vi "Drivetrain.vi"(10 "Duration":i64, 11 "rt fifo":refnum<k33>) -> ()   [LabVIEW 2015]
uses:
  Drive Metrics.ctl
  Drive States.ctl
  Copilot States.ctl
panel:
  in  "Drive Metrics":T1
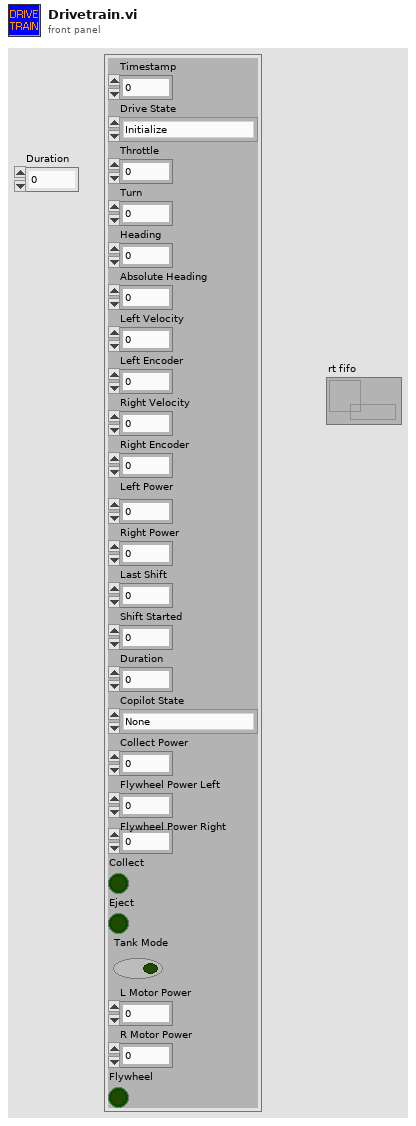
[diagram p1: front panel]
types:
  T1 = typedef "Drive Metrics.ctl" = cluster{"Timestamp":u32, "Drive State":T2, "Throttle":dbl, "Turn":dbl, "Heading":dbl, "Absolute Heading":dbl, "Left Velocity":dbl, "Left Encoder":dbl, "Right Velocity":dbl, "Right Encoder":dbl, "Left Power":dbl, "Right Power":dbl, "Last Shift":u32, "Shift Started":u32, "Duration":i64, "Copilot State":T3, "Collect Power":dbl, "Flywheel Power Left":dbl, "Flywheel Power Right":dbl, "Collect":bool, "Eject":bool, "Tank Mode":bool, "L Motor Power":dbl, "R Motor Power":dbl, "Flywheel":bool}
  T2 = typedef "Drive States.ctl" = enum16{"Initialize", "Low Gear", "Up Shift Begin", "Up Shifting", "Up Shift Delay", "High Gear", "Down Shift Begin", "Down Shifting", "Down Shift Delay"}
  T3 = typedef "Copilot States.ctl" = enum16{"None", "Lift collector", "Boulder to shooter", "Lifting collector", "Lifted Collector", "Collected", "Collecting", "Ejecting", "Dropping arm", "Boulder ready", "Shooter to angle", "Flywheel spin up", "Drop arm", "Flywheel ready"}
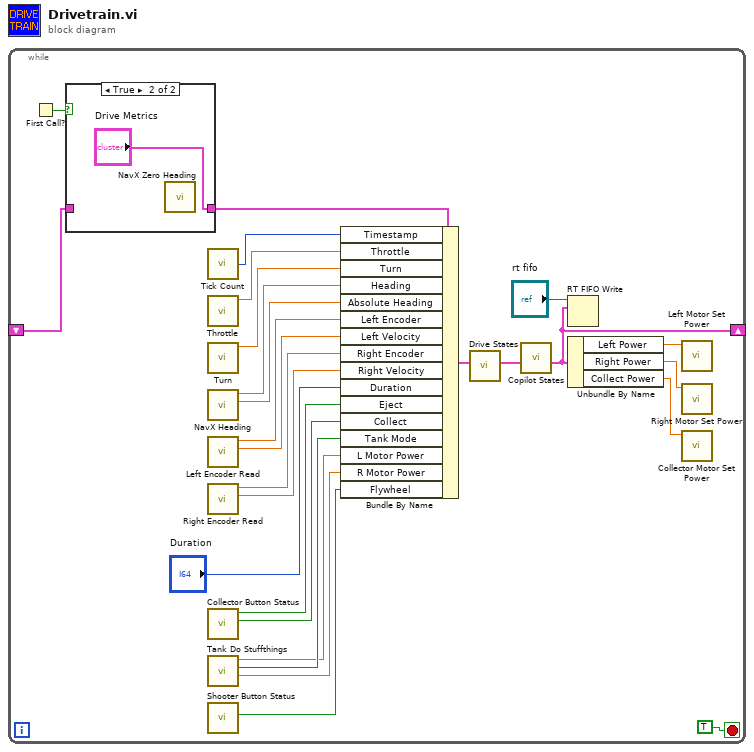
[diagram p0: block diagram]
diagram:
  n1 = while {
    shift-right: [w8] -> _
    shift-left: _ -> [w12]
    stop <- TRUE stop-if-true
    n2 = First Call?() -> (First Call?: T/F=w14:bool)
    n3 = case shown="True" w14 {
      tunnel: [w28 "Drive Metrics"] -> w13
      tunnel: w12 -> [w28 _]
      frame False {
      }
      frame True {
        n4 = call "NavX Zero Heading.vi"() -> ()  [unwired: 11 in, 1 out]
      }
    }
    n5 = call "Tick Count"() -> ("Tick Count(uSec)"=w10:u32)
    n6 = call "Throttle.vi"() -> ("throttle"=w26:dbl)  [unwired: 10 in, 1 out]
    n7 = call "Turn.vi"() -> ("turn"=w25:dbl)  [unwired: 10 in, 1 out]
    n8 = call "NavX Heading.vi"() -> ("Absolute Heading"=w17:dbl, "Heading"=w22:dbl)  [unwired: 9 in, 1 out]
    n9 = call "Left Encoder Read.vi"() -> ("Rate"=w16:dbl, "Distance"=w20:dbl)  [unwired: 7 in, 3 out]
    n10 = call "Right Encoder Read.vi"() -> ("Rate"=w15:dbl, "Distance"=w21:dbl)  [unwired: 7 in, 3 out]
    n11 = call "Collector Button Status.vi"() -> ("Collect"=w5:bool, "Eject"=w6:bool)  [unwired: 9 in, 1 out]
    n12 = call "Tank Do Stuffthings.vi"() -> ("R Motor Power"=w2:dbl, "Tank Mode"=w4:bool, "L Motor Power"=w3:dbl)  [unwired: 8 in, 1 out]
    n13 = call "Shooter Button Status.vi"() -> ("Flywheel"=w1:bool)  [unwired: 10 in, 1 out]
    n14 = Bundle By Name(cluster=w13, "Timestamp"=w10, "Throttle"=w26, "Turn"=w25, "Heading"=w22, "Absolute Heading"=w17, "Left Encoder"=w20, "Left Velocity"=w16, "Right Encoder"=w21, "Right Velocity"=w15, "Duration"="Duration", "Eject"=w6, "Collect"=w5, "Tank Mode"=w4, "L Motor Power"=w3, "R Motor Power"=w2, "Flywheel"=w1) -> (w18:T1)
    n15 = call "Drive States.vi"("Drive Metrics in"=w18) -> ("Drive Metrics out"=w9:T1)  [unwired: 10 in]
    n16 = call "Copilot States.vi"("Drive Metrics in"=w9) -> ("Drive Metrics out"=w8:T1)  [unwired: 10 in]
    n17 = RT FIFO Write(0:"rt fifo", 1:w8) -> ()  [unwired: 3 in, 4 out]
    n18 = Unbundle By Name(w8) -> ("Left Power"=w24:dbl, "Right Power"=w23:dbl, "Collect Power"=w7:dbl)
    n19 = call "Left Motor Set Power.vi"("Output"=w24) -> ()  [unwired: 10 in, 1 out]
    n20 = call "Right Motor Set Power.vi"("Output"=w23) -> ()  [unwired: 10 in, 1 out]
    n21 = call "Collector Motor Set Power.vi"("Output"=w7) -> ()  [unwired: 10 in, 1 out]
  }
